vi "CompareJointTorque.vi"() -> ()   [LabVIEW 2015]
uses:
  <vilib>/Utility/file.llb/Write To Spreadsheet File (DBL).vi
panel:
  out "Current File:":string
  out "Desired Torque":dbl[][](graph)
  out "Acutal Torque":dbl[][](graph)
  in  "File Name":string
  out "Total":i32
  out "Current":i32
  in  "pattern":string
  in  "Path":path
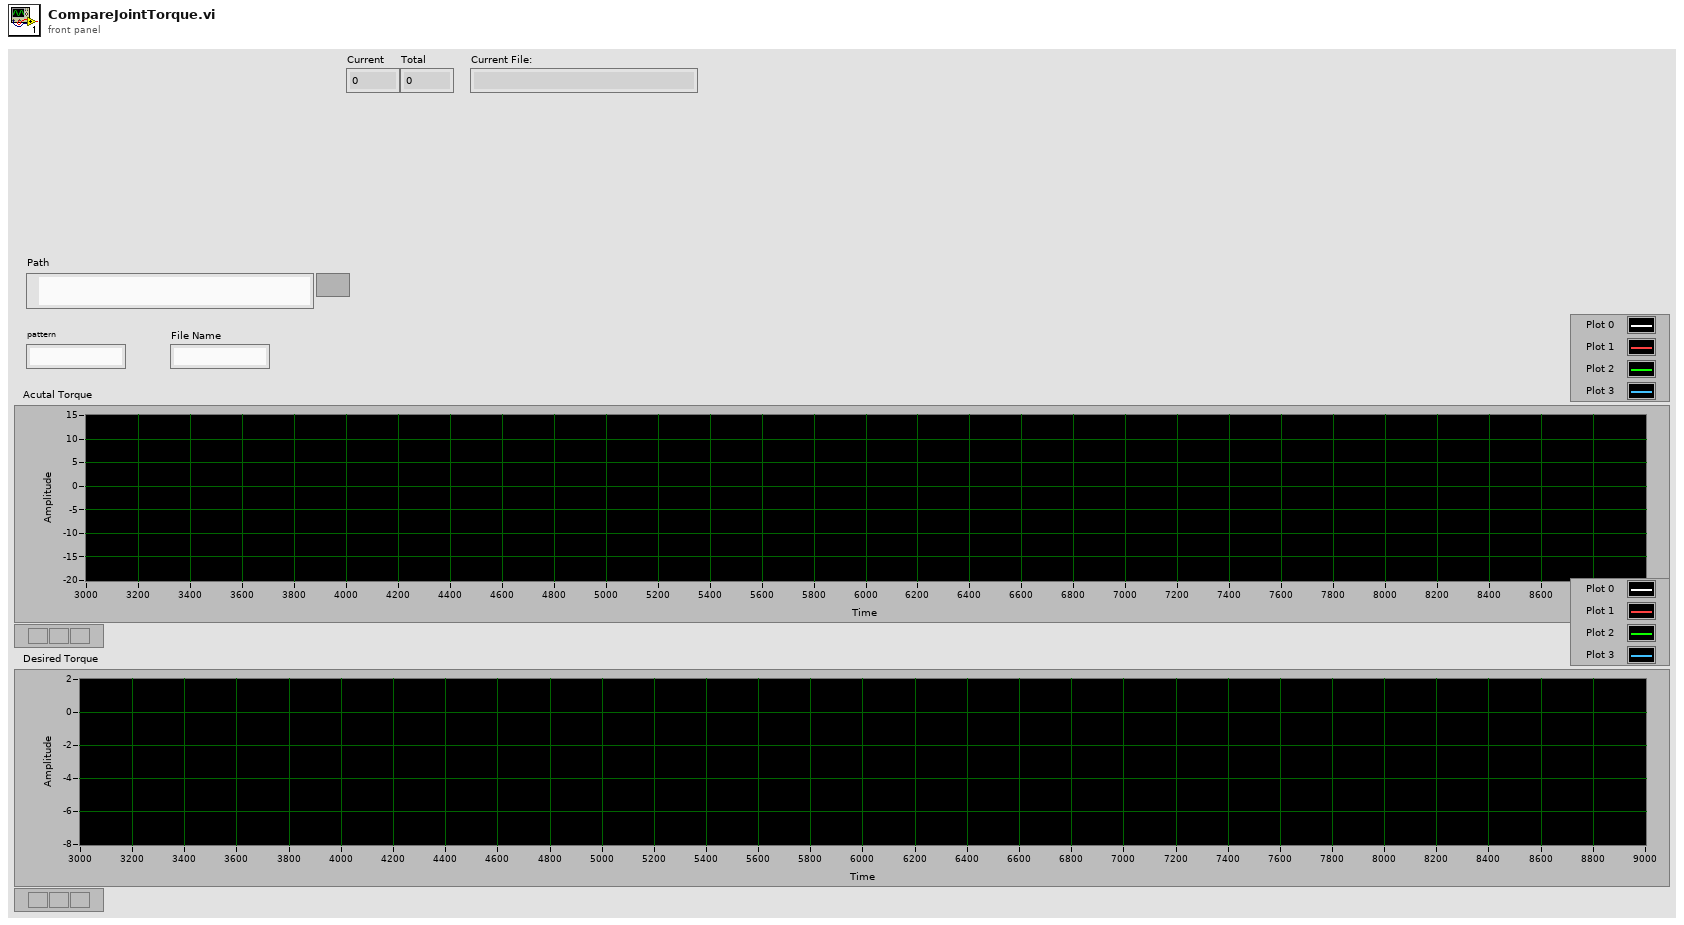
[diagram p1: front panel]
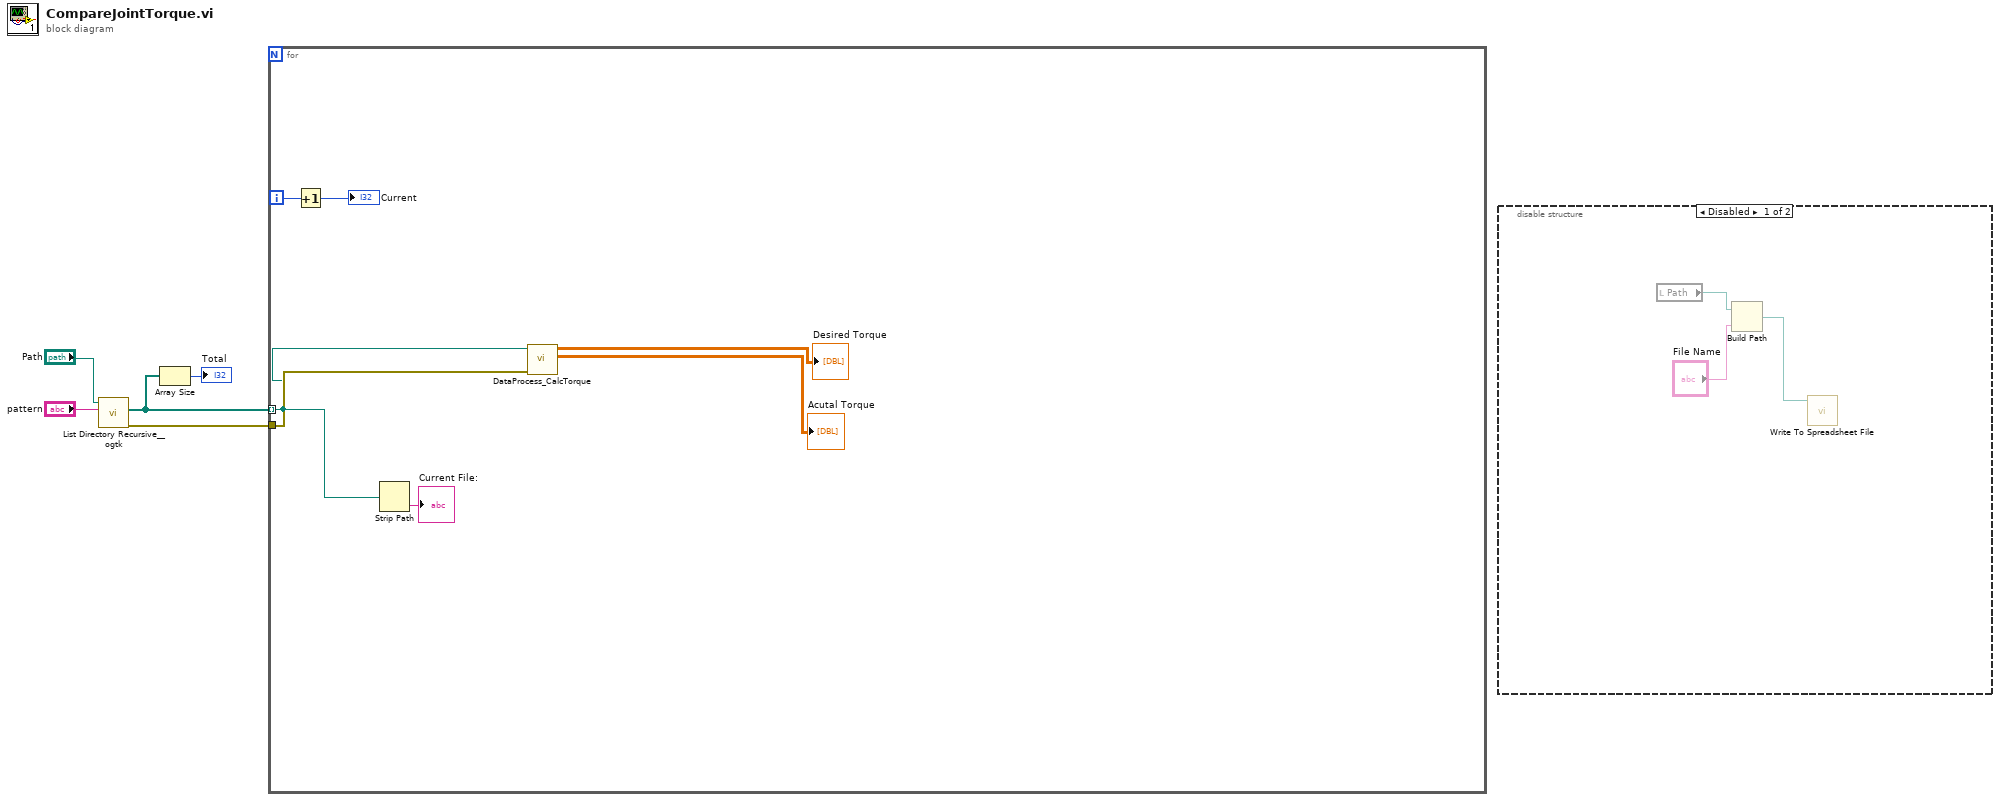
[diagram p0: block diagram]
diagram:
  n1 = call <userlib>:"List Directory Recursive__ogtk.vi"("pattern"="pattern", "Path"="Path") -> ("error out"=w3:errorcluster, "file paths"=w2:path[])  [unwired: 6 in, 2 out]
  n2 = Array Size(array=w2) -> (size(s)=→"Total":i32)
  n3 = for {
    tunnel: w2 -> [w9] mode=indexing
    tunnel: w3 -> [w10]
    i -> [w12]
    n4 = Increment(x=w12) -> (x+1=→"Current":i32)
    n5 = Strip Path(path=w9) -> (name=→"Current File:":string)  [unwired: 1 out]
    n6 = call "DataProcess_CalcTorque.vi"("error in (no error)"=w10, "Path"=w9) -> ("Acutal Torque"=→"Acutal Torque":dbl[][], "Desired Torque"=→"Desired Torque":dbl[][])  [unwired: 8 in]
  }
  n7 = disable-structure shown="Disabled" {
    frame Disabled {
      n8 = local read "Path"() -> (w16:path)
      n9 = Build Path(base path=w16, name or relative path="File Name") -> (appended path=w14:path)
      n10 = call-poly <vilib>:"Write To Spreadsheet File.vi"("file path (dialog if empty)"=w14) -> ("2D data"=w13:dbl[][])  [unwired: 6 in, 1 out]
    }
    frame Enabled {
    }
  }
